vi "To Byte Array (Characterization Data).vi"(1 "Characterization Data":T1 {"Frequencies [Hz]" format="%#_6p"}) -> (0 "byte array out":u8[](array[numeric]) format="%x")   [LabVIEW 2013]
uses:
  <instrlib>/ni579x/Config/v1/Shared/Types/ni579x Characterization Data.ctl
  <instrlib>/ni579x/Config/v1/Shared/Types/ni579x IQ Imbalance.ctl
  <instrlib>/ni579x/Config/v1/Shared/Types/ni579x Gain to Attenuation Mapping.ctl
  <instrlib>/ni579x/Config/v1/Shared/Conversions/To Byte Array (F32).vi
  <instrlib>/ni579x/Config/v1/Shared/Conversions/To Byte Array (U16).vi
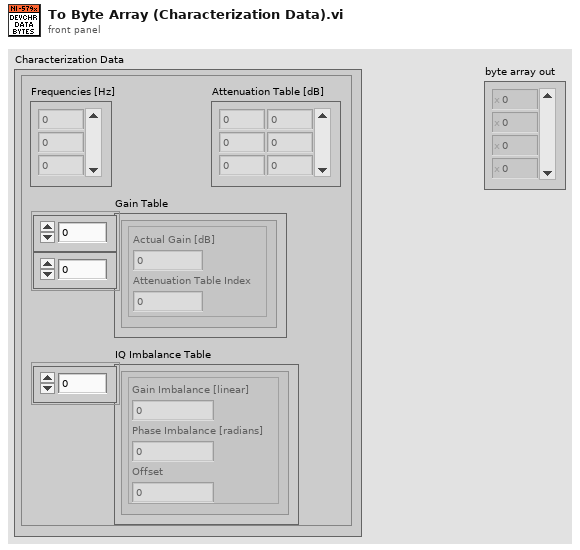
[diagram p1: front panel]
types:
  T1 = typedef "ni579x Characterization Data.ctl" = cluster{"Attenuation Table [dB]":dbl[][], "Frequencies [Hz]":dbl[], "IQ Imbalance Table":T2[], "Gain Table":T3[][]}
  T2 = typedef "ni579x IQ Imbalance.ctl" = cluster{"Gain Imbalance [linear]":dbl, "Phase Imbalance [radians]":dbl, "Offset":cdb}
  T3 = typedef "ni579x Gain to Attenuation Mapping.ctl" = cluster{"Actual Gain [dB]":dbl, "Attenuation Table Index":i32}
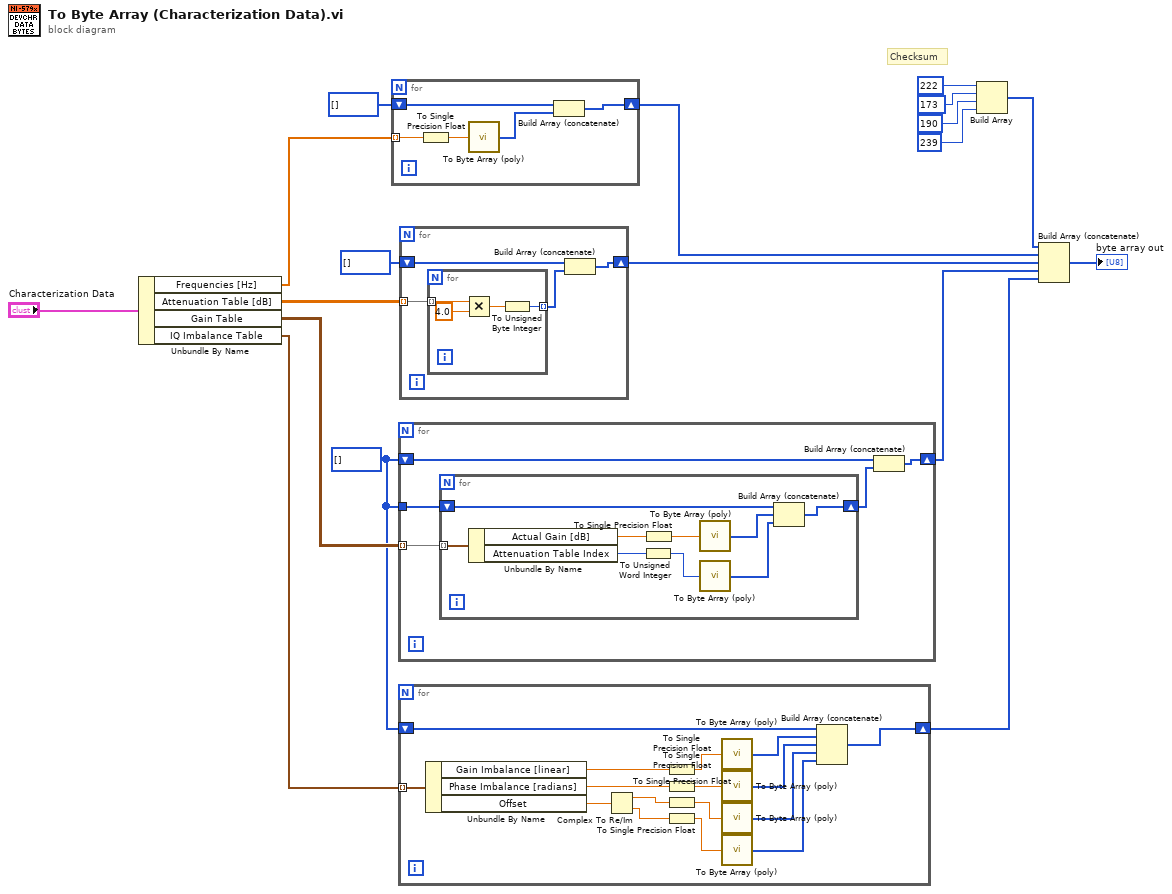
[diagram p0: block diagram]
diagram:
  w12 = u8[] []
  # "Checksum"
  n1 = Unbundle By Name("Characterization Data") -> ("Frequencies [Hz]"=w3:dbl[], "Attenuation Table [dB]"=w16:dbl[][], "Gain Table"=w14:T3[][], "IQ Imbalance Table"=w13:T2[])
  n2 = for {
    tunnel: w3 -> [w22] mode=indexing
    shift-right: [w20] -> w1
    shift-left: u8[] [] -> [w19]
    n3 = To Single Precision Float(number=w22) -> (single precision float=w23:sgl)
    n4 = call-poly <instrlib>:"To Byte Array (poly).vi"("element in"=w23) -> ("byte array out"=w21:u8[])
    n5 = Build Array (concatenate)(w19, w21) -> (w20:u8[])
  }
  n6 = for {
    tunnel: w14 -> [w28] mode=indexing
    shift-right: [w26] -> w10
    shift-left: w12 -> [w25]
    tunnel: w12 -> [w24]
    n7 = for {
      tunnel: w28 -> [w37] mode=indexing
      shift-right: [w30] -> w27
      shift-left: w24 -> [w29]
      n8 = Unbundle By Name(w37) -> ("Actual Gain [dB]"=w36:dbl, "Attenuation Table Index"=w35:i32)
      n9 = To Unsigned Word Integer(number=w35) -> (unsigned 16bit integer=w33:u16)
      n10 = To Single Precision Float(number=w36) -> (single precision float=w34:sgl)
      n11 = call-poly <instrlib>:"To Byte Array (poly).vi"("element in"=w34) -> ("byte array out"=w32:u8[])
      n12 = call-poly <instrlib>:"To Byte Array (poly).vi"("element in"=w33) -> ("byte array out"=w31:u8[])
      n13 = Build Array (concatenate)(w29, w32, w31) -> (w30:u8[])
    }
    n14 = Build Array (concatenate)(w25, w27) -> (w26:u8[])
  }
  n15 = for {
    tunnel: w13 -> [w53] mode=indexing
    shift-right: [w39] -> w9
    shift-left: w12 -> [w38]
    n16 = Unbundle By Name(w53) -> ("Gain Imbalance [linear]"=w51:dbl, "Phase Imbalance [radians]"=w50:dbl, "Offset"=w52:cdb)
    n17 = Complex To Re/Im(x + iy=w52) -> (x=w49:dbl, y=w48:dbl)
    n18 = To Single Precision Float(number=w51) -> (single precision float=w47:sgl)
    n19 = To Single Precision Float(number=w50) -> (single precision float=w46:sgl)
    n20 = To Single Precision Float(number=w49) -> (single precision float=w45:sgl)
    n21 = To Single Precision Float(number=w48) -> (single precision float=w44:sgl)
    n22 = call-poly <instrlib>:"To Byte Array (poly).vi"("element in"=w47) -> ("byte array out"=w40:u8[])
    n23 = call-poly <instrlib>:"To Byte Array (poly).vi"("element in"=w46) -> ("byte array out"=w41:u8[])
    n24 = call-poly <instrlib>:"To Byte Array (poly).vi"("element in"=w45) -> ("byte array out"=w42:u8[])
    n25 = call-poly <instrlib>:"To Byte Array (poly).vi"("element in"=w44) -> ("byte array out"=w43:u8[])
    n26 = Build Array (concatenate)(w38, w40, w41, w42, w43) -> (w39:u8[])
  }
  n27 = for {
    tunnel: w16 -> [w57] mode=indexing
    shift-right: [w55] -> w11
    shift-left: u8[] [] -> [w54]
    n28 = for {
      tunnel: w57 -> [w61] mode=indexing
      tunnel: [w58] -> w56 mode=indexing
      n29 = Multiply(x=w61, y=4.0) -> (x*y=w59:dbl)
      n30 = To Unsigned Byte Integer(number=w59) -> (unsigned 8bit integer=w58:u8)
    }
    n31 = Build Array (concatenate)(w54, w56) -> (w55:u8[])
  }
  n32 = Build Array(u8 222 ("element"), u8 173 ("element"), u8 190 ("element"), u8 239 ("element")) -> (w4:u8[])
  n33 = Build Array (concatenate)(w4, w1, w11, w10, w9) -> (→"byte array out":u8[])
